vi "edit_variant_name.vi"(7 "update variant":string, 8 "error in (no error)":errorcluster, 9 "Input values":T1, 10 "Delete variant":string, 11 "configuration file path":path) -> (0 "error out":errorcluster, 3 "file path":path)   [LabVIEW 2021]
uses:
  <vilib>/Utility/config.llb/Write Key (String).vi
  <vilib>/Utility/config.llb/NI_LVConfig.lvlib
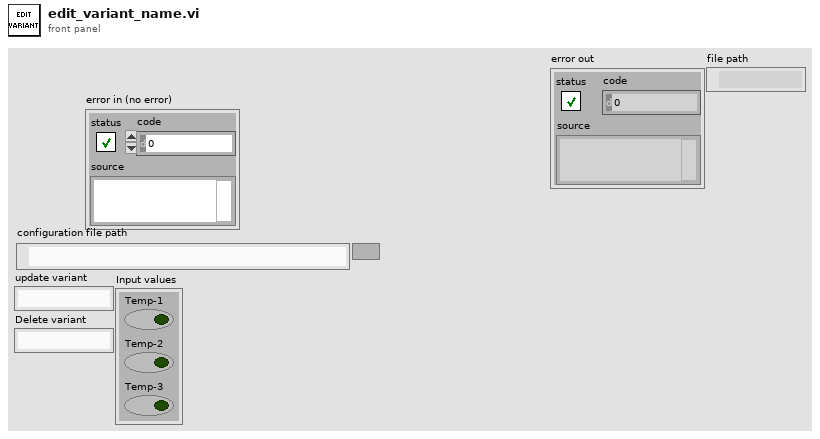
[diagram p1: front panel]
types:
  T1 = cluster{"Temp-1":bool, "Temp-2":bool, "Temp-3":bool}
  T2 = typedef "NI_LVConfig.lvlib/Config Data RefNum.ctl" = refnum<k1>
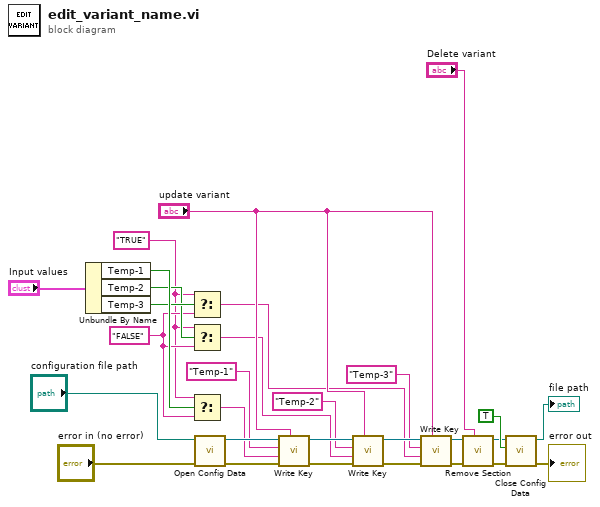
[diagram p0: block diagram]
diagram:
  w13 = "FALSE"
  w12 = "TRUE"
  n1 = Unbundle By Name("Input values") -> ("Temp-1"=w16:bool, "Temp-2"=w14:bool, "Temp-3"=w15:bool)
  n2 = Select(t=w12, s=w15, f=w13) -> (s? t:f=w9:string)
  n3 = Select(t=w12, s=w14, f=w13) -> (s? t:f=w10:string)
  n4 = Select(t=w12, s=w16, f=w13) -> (s? t:f=w11:string)
  n5 = call <vilib>:"Open Config Data.vi"("error in (no error)"="error in (no error)", "configuration file path"="configuration file path") -> ("error out"=w25:errorcluster, "refnum"=w24:T2)  [unwired: 7 in, 1 out]
  n6 = call-poly <vilib>:"Write Key.vi"("section"="update variant", "error in (no error)"=w25, "value"=w11, "key"="Temp-1", "refnum"=w24) -> ("error out"=w20:errorcluster, "refnum out"=w18:T2)  [unwired: 4 in, 1 out]
  n7 = call-poly <vilib>:"Write Key.vi"("section"="update variant", "error in (no error)"=w20, "value"=w10, "key"="Temp-2", "refnum"=w18) -> ("error out"=w19:errorcluster, "refnum out"=w17:T2)  [unwired: 4 in, 1 out]
  n8 = call-poly <vilib>:"Write Key.vi"("section"="update variant", "error in (no error)"=w19, "value"=w9, "key"="Temp-3", "refnum"=w17) -> ("error out"=w3:errorcluster, "refnum out"=w5:T2)  [unwired: 4 in, 1 out]
  n9 = call <vilib>:"Remove Section.vi"("section"="Delete variant", "error in (no error)"=w3, "refnum"=w5) -> ("error out"=w2:errorcluster, "refnum out"=w4:T2)  [unwired: 6 in, 1 out]
  n10 = call <vilib>:"Close Config Data.vi"("error in (no error)"=w2, "write file if changed (T)"=TRUE, "refnum"=w4) -> ("error out"=→"error out":errorcluster, "file path"=→"file path":path)  [unwired: 7 in]
